vi "Simple_2D_AA_SS3_filter.vi"(8 "error in (no error)":errorcluster, 10 "Image Pixels (U32)":u32[][](array[numeric]), 11 "Refnum in":T1) -> (0 "error out":errorcluster, 3 "Refnum out":T1)   [LabVIEW 2018]
uses:
  <vilib>/vision/Image Controls.llb/IMAQ Image.ctl
  <vilib>/Analysis/2dsp.llb/2D Convolution (DBL).vi
  <vilib>/Analysis/NI_AALPro.lvlib
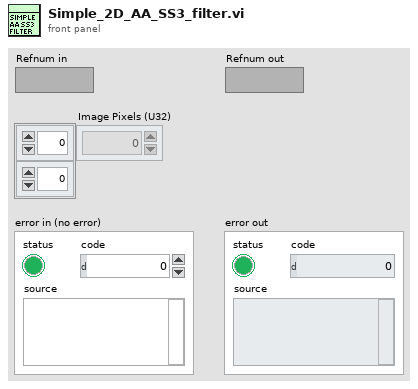
[diagram p1: front panel]
types:
  T1 = typedef "IMAQ Image.ctl" = refnum<image>
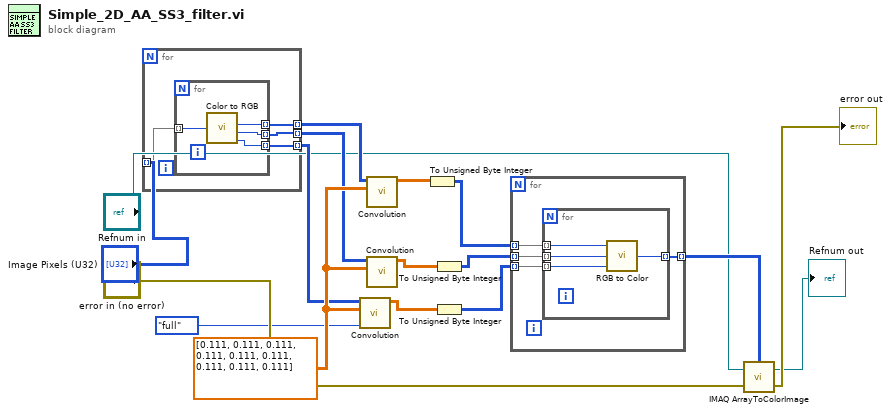
[diagram p0: block diagram]
diagram:
  w10 = dbl[][] [[0.111, 0.111, 0.111], [0.111, 0.111, 0.111], [0.111, 0.111, 0.111]] ("Y")
  n1 = for {
    tunnel: "Image Pixels (U32)" -> [w21] mode=indexing
    tunnel: [w20] -> w7 mode=indexing
    tunnel: [w19] -> w8 mode=indexing
    tunnel: [w18] -> w9 mode=indexing
    n2 = for {
      tunnel: w21 -> [w25] mode=indexing
      tunnel: [w24] -> w20 mode=indexing
      tunnel: [w23] -> w19 mode=indexing
      tunnel: [w22] -> w18 mode=indexing
      n3 = call <vilib>:"Color to RGB.vi"("Color"=w25) -> ("R"=w24:u8, "G"=w23:u8, "B"=w22:u8)  [unwired: 1 out]
    }
  }
  n4 = call-poly <vilib>:"Convolution.vi"("output size"=enum32{"full", "size X", "compact"}."full", "Y"=w10, "X"=w9) -> ("X * Y"=w13:dbl[][])  [unwired: 7 in, 1 out]
  n5 = call-poly <vilib>:"Convolution.vi"("Y"=w10, "X"=w7) -> ("X * Y"=w11:dbl[][])  [unwired: 8 in, 1 out]
  n6 = call-poly <vilib>:"Convolution.vi"("Y"=w10, "X"=w8) -> ("X * Y"=w12:dbl[][])  [unwired: 8 in, 1 out]
  n7 = To Unsigned Byte Integer(number=w11) -> (unsigned 8bit integer=w14:u8[][])
  n8 = To Unsigned Byte Integer(number=w12) -> (unsigned 8bit integer=w15:u8[][])
  n9 = To Unsigned Byte Integer(number=w13) -> (unsigned 8bit integer=w16:u8[][])
  n10 = for {
    tunnel: w14 -> [w29] mode=indexing
    tunnel: w15 -> [w28] mode=indexing
    tunnel: w16 -> [w27] mode=indexing
    tunnel: [w26] -> w17 mode=indexing
    n11 = for {
      tunnel: w29 -> [w33] mode=indexing
      tunnel: w28 -> [w32] mode=indexing
      tunnel: w27 -> [w31] mode=indexing
      tunnel: [w30] -> w26 mode=indexing
      n12 = call <vilib>:"RGB to Color.vi"("B"=w31, "G"=w32, "R"=w33) -> ("Color"=w30:u32)
    }
  }
  n13 = call "IMAQ ArrayToColorImage"("Image Pixels (U32)"=w17, "Image"="Refnum in", "error in (no error)"="error in (no error)") -> ("Image Out"=→"Refnum out":T1, "error out"=→"error out":errorcluster)  [unwired: 2 in]
